vi "ProdaNG.IdentifyMe.vi"(6 "wabcoNumber":string, 7 "systemName":string, 8 "error in":errorcluster, 9 "processSequence":i32, 10 "processId":i32, 11 "dbHandleIn":i32) -> (0 "error out":errorcluster, 2 "Identification":T1, 3 "dbHandle":i32)   [LabVIEW 2016]
doc: "This function serves for identifying a system, if for example, the name and the Wabco Number of the tested part, or the process id and the sequential number in a process are known. \nParameter:\nhandle is an Integer, which is returned by the function Login() at the creation of a new connection.\nsystemName is the name of the system, as it is deposited in the database. If unknown, NULL must be passed.\nwabcoNumber is a known Wabco number in the database. If unknown, NULL must be passed.\nprocessSequence is the sequential Number in the process. If unknown, 0 must be passed.\nprocessId is the according process id. If unknown, 0 must be passed.\n\nmyIdent is a pointer on an identification structure, if the returncode is 0. The structure must be defined in the calling program. The function tries to identify the system definitely under the aid of the passed parameter, in order to return the resulting id's in MyIdent.\n\nThe function tries to identify the system from the following combinations of the parameter:\nsystemName, \nprocessId, \nsystemName and wabcoNumber, \nprocessId and processSequence \nor from all 4 parameter.\nThe more parameters are set, the bigger is the chance, that the system can be identified.\nReturncodes:\n0 No error\n< 0 ORACLE Error Code\n6 (ERROR_INVALID_HANDLE) in case of an invalid handle\n232 (ERROR_NO_DATA) in case that the system cannot be identified definitely."
uses:
  Controls/ProdaNG.Identification.ctl
  prodllNG.dll
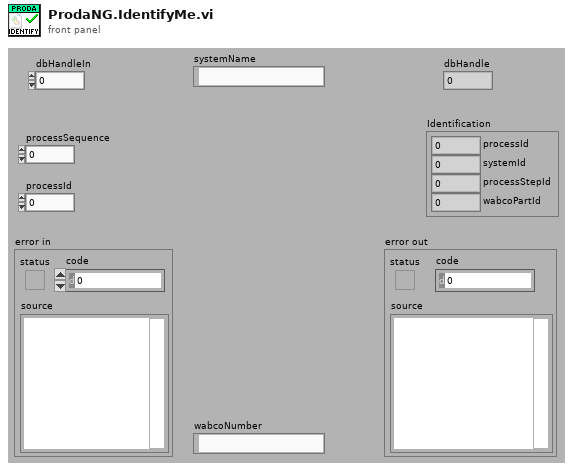
[diagram p1: front panel]
types:
  T1 = typedef "ProdaNG.Identification.ctl" = cluster{"processId":i32, "systemId":i32, "processStepId":i32, "wabcoPartId":i32}
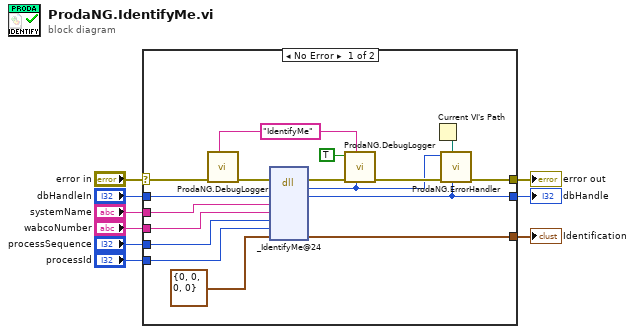
[diagram p0: block diagram]
diagram:
  n1 = case shown="No Error" "error in" {
    selector: "error in" -> [w21 w28]
    tunnel: [w25 w28] -> w8
    tunnel: [w16 w27] -> w7
    tunnel: "dbHandleIn" -> [w15 w27]
    tunnel: [w14 _] -> w5
    tunnel: "systemName" -> [w13 _]
    tunnel: "wabcoNumber" -> [w12 _]
    tunnel: "processSequence" -> [w11 _]
    tunnel: "processId" -> [w10 _]
    frame No Error {
      w23 = "IdentifyMe" ("cmd")
      n2 = call "ProdaNG.DebugLogger.vi"("cmd"=w23, "error in (no error)"=w21) -> ("error out"=w20:errorcluster)  [unwired: 9 in]
      n3 = dll-call lib="D:/svn/LineTraceSystem/SOFTWARE/sources/Database/ProdaNG/prodllNG.dll" fn="_IdentifyMe@24" ("ProDll.dll:Login")(error in=w20, "dbHandle"=w15, "systemName"=w13, "wabcoNumber"=w12, "processSequence"=w11, "processId"=w10, "Identification"=T1 {"processId"=0, "systemId"=0, "processStepId"=0, "wabcoPartId"=0}) -> (error out=w19:errorcluster, w17:i32, "dbHandle"=w16:i32, "Identification"=w14:T1)  [unwired: 6 in, 1 out]
      n4 = call "ProdaNG.DebugLogger.vi"("return type"=w17, "cmd"=w23, "error in (no error)"=w19, "done? (F)"=TRUE) -> ("error out"=w18:errorcluster)  [unwired: 7 in]
      n5 = Current VI's Path() -> (path=w24:path)
      n6 = call "ProdaNG.ErrorHandler.vi"("dbHandleIn"=w16, "Path"=w24, "error in"=w18, "output_parameter"=w17) -> ("error out"=w25:errorcluster)  [unwired: 7 in]
    }
    frame Error {
    }
  }
  "error out" <- w8
  "dbHandle" <- w7
  "Identification" <- w5
